vi "LCR_BK891_SoftFP.vi"(0 "reference in":refnum<class "LCR_BK891.lvclass">, 2 "Floating":bool, 5 "error in (no error)":errorcluster) -> (14 "reference out":refnum<class "LCR_BK891.lvclass">, 19 "error out":errorcluster)   [LabVIEW 2022 SP3, in "LCR_BK891.lvlib" / "LCR_BK891.lvclass"]
uses:
  LCR_BK891.lvclass
  Components/ViPER.lvlibp/ViPER.lvclass
  C:/Projects/Medulla/ViPER/Examples/Flux_Capacitor_Tester/Components/ViPER.lvlibp/ViPER.lvclass
panel:
  in  "Speed":u16(ring) caption="Ring" items=["Slow"=1, "Fast"=2]
  in  "Range":u16(ring) caption="Ring" items=["Hold", "Auto"]
  in  "Function":u16(ring) caption="Ring" items=["Cs-Q", "Cs-D", "Cs-R", "Cp-Q", "Cp-D", "Cp-R", "Cp-G", "Ls-Q", "Ls-D", "Ls-R", "Lp-Q", "Lp-D", "Lp-R", "Lp-G", "Z-th", "Y-th", "R-X", "G-B", "DCR"]
  in  "Level":u8(ring) caption="Ring" items=["0.5Vrms", "1Vrms"]
  in  "Frequency":dbl caption="Numeric"
  out "Primary Reading":dbl caption="Numeric"
  out "Secondary Reading":dbl caption="Numeric"
  in  "Measure":bool
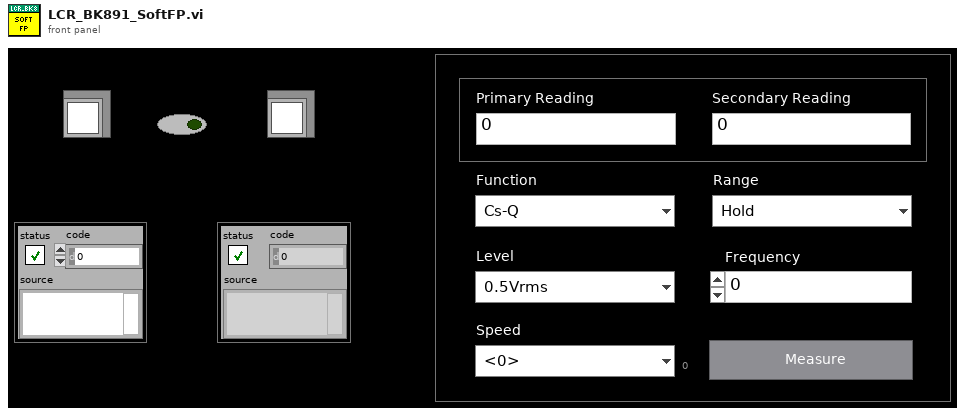
[diagram p1: front panel]
types:
  T1 = enum32{"Invalid", "Standard", "Closed", "Hidden", "Minimized", "Maximized"}
  T2 = typedef "LCR_BK891.lvlib/LCR_BK891.lvclass/ObjectAttributes.ctl" = cluster{"Config":T3, "VISA Ref":refnum<visa-resource-name>, "Function":u16, "Range":u16, "Measurement Speed":u16, "Signal Frequency":dbl, "Signal Level":u8, "Measured Primary Reading":dbl, "Measured Secondary Reading":dbl}
  T3 = typedef "LCR_BK891.lvlib/LCR_BK891.lvclass/Config.ctl" = cluster{"VISA":refnum<visa-resource-name>}
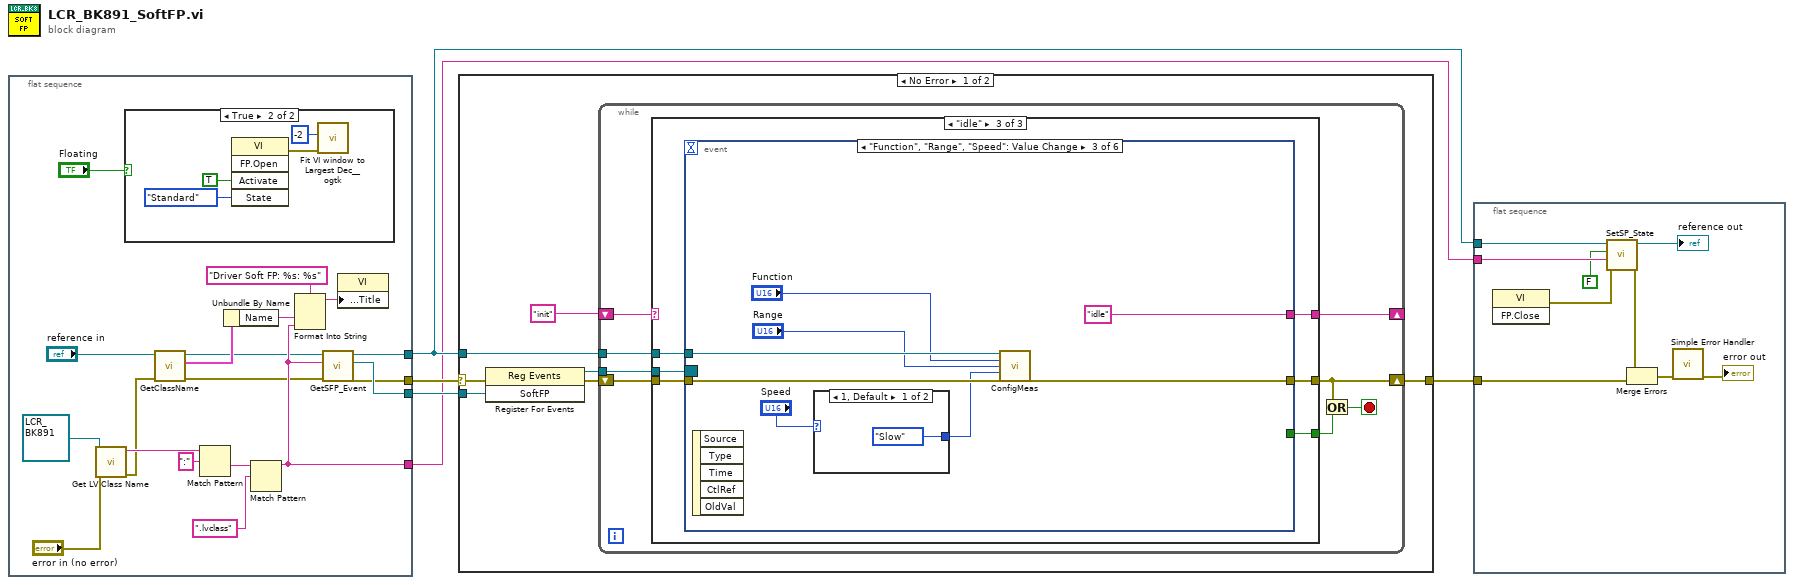
[diagram p0: block diagram]
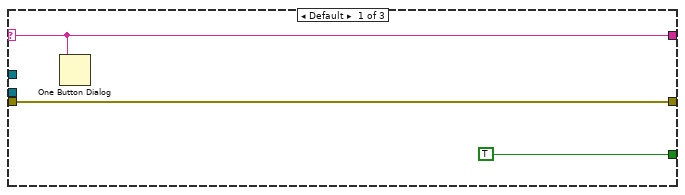
[diagram p3: hidden frame]
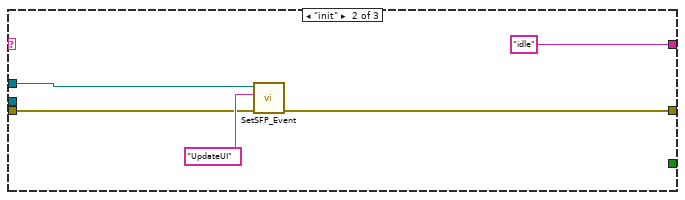
[diagram p4: hidden frame]
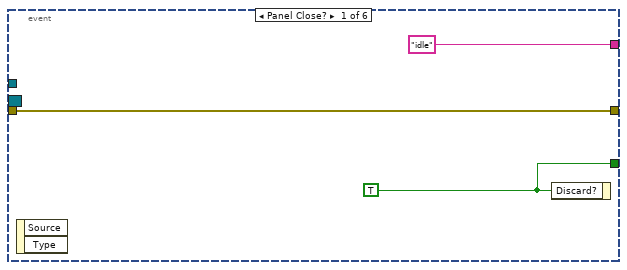
[diagram p5: hidden frame]
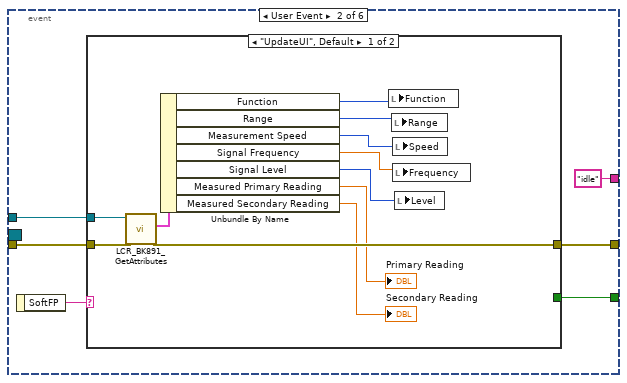
[diagram p6: hidden frame]
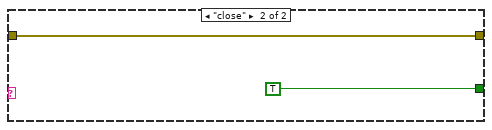
[diagram p7: hidden frame]
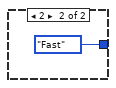
[diagram p8: hidden frame]
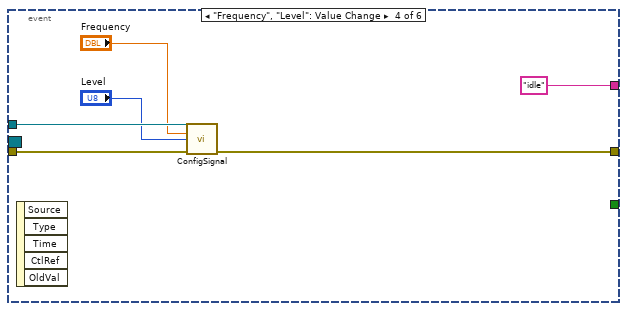
[diagram p9: hidden frame]
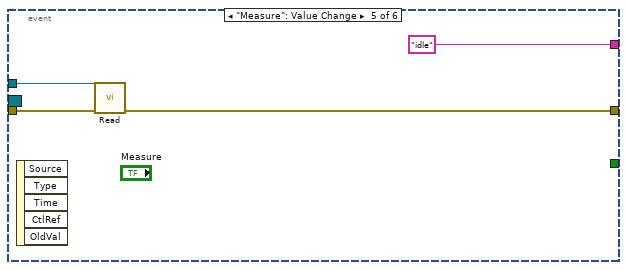
[diagram p10: hidden frame]
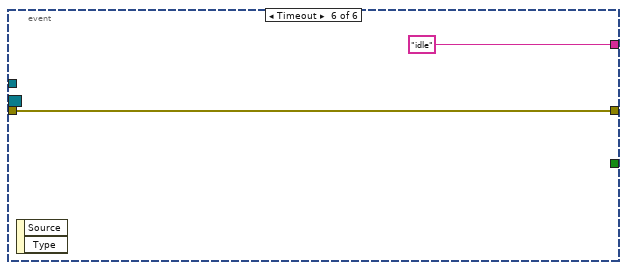
[diagram p11: hidden frame]
diagram:
  n1 = flat-sequence {
    tunnel: [w21] -> w5
    tunnel: [w20] -> w2
    tunnel: [w24] -> w3
    tunnel: [w12] -> w1
    frame #0 {
      n2 = call <vilib>:"Get LV Class Name.vi"("error in (no error)"="error in (no error)", "object"=refnum<class "LCR_BK891.lvclass"> refnum ("reference")) -> ("error out"=w11:errorcluster, "class name"=w17:string)  [unwired: 8 in]
      n3 = case shown="True" "Floating" {
        frame False {
        }
        frame True {
          n4 = invoke class="VI" method="FP.Open"("Activate"=TRUE ("Activate?"), "State"=T1."Standard") -> (error out=w25:errorcluster)  [unwired: 3 in, 4 out]
          n5 = call <userlib>:"Fit VI window to Largest Dec__ogtk.vi"("error in (no error)"=w25, "border spacing (2 px)"=-2) -> ()  [unwired: 4 in, 2 out]
        }
      }
      n6 = call "GetClassName.vi"("error in (no error)"=w11, "reference in"="reference in") -> ("error out"=w10:errorcluster, "Details"=w9:cluster{"Name":string, "Class":string}, "reference out"=w7:refnum<class "LCR_BK891.lvclass">)  [unwired: 7 in]
      n7 = Match Pattern(string=w17, regular expression=":") -> (after substring=w15:string)  [unwired: 1 in, 3 out]
      n8 = Unbundle By Name(w9) -> ("Name"=w19:string)
      n9 = Match Pattern(string=w15, regular expression=".lvclass") -> (before substring=w12:string)  [unwired: 1 in, 3 out]
      n10 = Format Into String(format string="Driver Soft FP: %s: %s", w19, w12) -> (resulting string=w23:string)  [unwired: 2 in, 1 out]
      n11 = call-dynamic "GetSFP_Event.vi"("error in (no error)"=w10, "Ancestor"=w12, "reference in"=w7) -> ("error out"=w21:errorcluster, "SoftFP"=w24:refnum<user-event>, "reference out"=w20:refnum<class "LCR_BK891.lvclass">)  [unwired: 6 in]
      n12 = property class="VI"("Front Panel.Title"=w23) -> ()  [unwired: 2 in, 2 out]
    }
  }
  n13 = case shown="No Error" w5 {
    selector: w5 -> [w33 w102]
    tunnel: [w29 w102] -> w4
    tunnel: w2 -> [w30 _]
    tunnel: w3 -> [w35 _]
    frame No Error {
      n14 = register-events(error in=w33, w35) -> (reference out=w34:refnum<event-registration>, error out=w32:errorcluster)  [unwired: 1 in]
      n15 = while {
        shift-right: [w40] -> w29
        shift-left: w32 -> [w43]
        tunnel: w34 -> [w42]
        tunnel: w30 -> [w41]
        shift-right: [w36] -> _
        shift-left: "init" -> [w37]
        stop <- w39 stop-if-true
        n16 = case shown="\"idle\"" w37 {
          selector: w37 -> [w44 _ _]
          tunnel: w43 -> [w45 w48 w57]
          tunnel: w42 -> [_ _ w56]
          tunnel: w41 -> [_ w47 w55]
          tunnel: [w45 w49 w54] -> w40
          tunnel: [TRUE ("Discard?") _ w53] -> w38
          tunnel: [w44 "idle" w52] -> w36
          frame Default {
            n17 = One Button Dialog(message=w44) -> ()  [unwired: 1 in, 1 out]
          }
          frame "init" {
            n18 = call-dynamic "SetSFP_Event.vi"("error in (no error)"=w48, "msg"="UpdateUI", "reference in"=w47) -> ("error out"=w49:errorcluster)  [unwired: 7 in, 1 out]
          }
          frame "idle" {
            n19 = event shown="[2] \"Function\", \"Range\", \"Speed\": Value Change" {
              selector: w56 -> [_ _ _ _ _ _]
              dyn-events: _ -> [_ _ _ _ _ _]
              timeout: _ -> [_ _ _ _ _ _]
              tunnel: w57 -> [w60 w66 w87 w95 w98 w101]
              tunnel: [w60 w64 w86 w93 w96 w101] -> w54
              tunnel: [w59 w63 _ _ _ _] -> w53
              tunnel: w55 -> [_ w61 w85 w94 w97 _]
              tunnel: ["idle" "idle" "idle" "idle" "idle" "idle"] -> w52
              event Panel Close? {
                w59 = TRUE ("Discard?")
                n20 = event-data() -> ()  [unwired: 1 in, 2 out]
                n21 = event-data("Discard?"=w59) -> ()  [unwired: 1 in, 1 out]
              }
              event User Event {
                n22 = event-data() -> ("SoftFP"=w65:string)  [unwired: 1 in]
                n23 = case shown="\"UpdateUI\", Default" w65 {
                  tunnel: w66 -> [w76 w79]
                  tunnel: [w77 w79] -> w64
                  tunnel: [_ TRUE ("Discard?")] -> w63
                  tunnel: w61 -> [w75 _]
                  frame "UpdateUI", Default {
                    n24 = call "LCR_BK891_GetAttributes.vi"("error in (no error)"=w76, "reference in"=w75) -> ("error out"=w77:errorcluster, "Data"=w74:T2)  [unwired: 6 in, 2 out]
                    n25 = Unbundle By Name(w74) -> ("Function"=w71:u16, "Range"=w70:u16, "Measurement Speed"=w69:u16, "Signal Frequency"=w68:dbl, "Signal Level"=w67:u8, "Measured Primary Reading"=→"Primary Reading":dbl, "Measured Secondary Reading"=→"Secondary Reading":dbl)
                    n26 = local write "Function"(w71) -> ()
                    n27 = local write "Range"(w70) -> ()
                    n28 = local write "Speed"(w69) -> ()
                    n29 = local write "Frequency"(w68) -> ()
                    n30 = local write "Level"(w67) -> ()
                  }
                  frame "close" {
                  }
                }
              }
              event "Function", "Range", "Speed": Value Change {
                n31 = event-data() -> ()  [unwired: 1 in, 5 out]
                n32 = case shown="1, Default" "Speed" {
                  tunnel: [enum16{"Slow", "Fast"}."Slow" ("Meas_Speed") enum16{"Slow", "Fast"}."Fast" ("Meas_Speed")] -> w80
                  frame 1, Default {
                  }
                  frame 2 {
                  }
                }
                n33 = call-dynamic "ConfigMeas.vi"("reference in"=w85, "Function (4: Cp-D)"="Function", "Range (1:Auto)"="Range", "Meas_Speed"=w80, "error in (no error)"=w87) -> ("error out"=w86:errorcluster)  [unwired: 9 in, 1 out]
              }
              event "Frequency", "Level": Value Change {
                n34 = event-data() -> ()  [unwired: 1 in, 5 out]
                n35 = call-dynamic "ConfigSignal.vi"("reference in"=w94, "Signal Frequency (1000 Hz)"="Frequency", "Signal Level (0:0.5 Vrms)"="Level", "error in (no error)"=w95) -> ("error out"=w93:errorcluster)  [unwired: 10 in, 1 out]
              }
              event "Measure": Value Change {
                n36 = event-data() -> ()  [unwired: 1 in, 5 out]
                n37 = call-dynamic "Read.vi"("reference in"=w97, "error in (no error)"=w98) -> ("error out"=w96:errorcluster)  [unwired: 10 in, 3 out]
              }
              event Timeout {
                n38 = event-data() -> ()  [unwired: 1 in, 2 out]
              }
            }
          }
        }
        n39 = Or(x=w40, y=w38) -> (x .or. y?=w39:bool)
      }
    }
    frame Error {
    }
  }
  n40 = flat-sequence {
    tunnel: w4 -> [w109]
    tunnel: w2 -> [w104]
    tunnel: w1 -> [w106]
    frame #0 {
      n41 = invoke class="VI" method="FP.Close"() -> (error out=w108:errorcluster)  [unwired: 3 in, 2 out]
      n42 = call "SetSP_State.vi"("error in (no error)"=w108, "Ancestor"=w106, "SP Open"=FALSE, "reference in"=w104) -> ("error out"=w107:errorcluster, "reference out"=→"reference out":refnum<class "LCR_BK891.lvclass">)  [unwired: 6 in]
      n43 = Merge Errors(w107, w109) -> (w111:errorcluster)
      n44 = call <vilib>:"Simple Error Handler.vi"("error in (no error)"=w111) -> ("error out"=→"error out":errorcluster)  [unwired: 4 in, 4 out]
    }
  }
